vi "Close.vi"(8 "error in (no error)":errorcluster, 11 "Message Queue in":refnum<class "Message Queue.lvclass">) -> (0 "error out":errorcluster, 3 "Message Queue out":refnum<class "Message Queue.lvclass">)   [LabVIEW 2027, in "Messaging.lvlib" / "Message Queue.lvclass"]
uses:
  Message Queue.lvclass
  Message Queue.lvclass/Message Queue.ctl
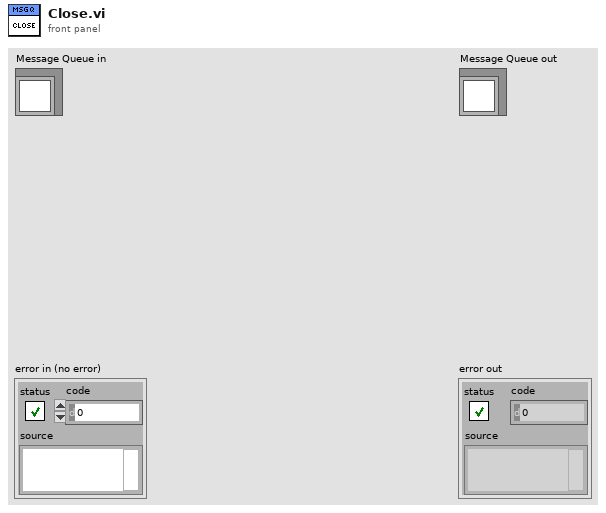
[diagram p1: front panel]
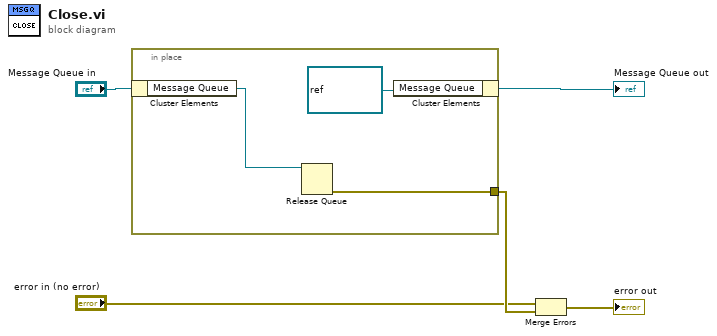
[diagram p0: block diagram]
diagram:
  n1 = in-place {
    in-place-border: [w7] -> w5
    n2 = in-place-cluster #1("Message Queue in") -> ("Message Queue"=w8:refnum<queue>)
    n3 = Release Queue(queue=w8) -> (error out=w7:errorcluster)  [unwired: 2 in, 2 out]
    n4 = in-place-cluster #1("Message Queue"=refnum<queue> refnum) -> (→"Message Queue out":refnum<class "Message Queue.lvclass">)
  }
  n5 = Merge Errors("error in (no error)", w5) -> (→"error out":errorcluster)
